vi "Teleop.vi"(10 "Match Info":T1={"Autonomous Elapsed Seconds"=0.0, "TeleOp Elapsed Seconds"=0.0, "Disabled Elapsed Seconds"=0.0, "Visited Autonomous"=FALSE, "Visited TeleOp"=FALSE, "Visited Disabled"=FALSE, "Autonomous Settings"={"Autonomous Style"=enum."Independent", "VI Refnum"=refnum}}, 11 "Call Context":T2) -> ()   [LabVIEW 2018]
doc: "This VI is called for each TeleOp packet received from the DS where the robot is not disabled. It is often used to read from the joysticks and update I/O or to update setpoints for timed control loops. It should complete and return within 20 milliseconds or it may miss DS packets."
uses:
  <vilib>/Rock Robotics/WPI/DriverStation/WPI_DriverStationDerivedRobotMode.ctl
  <vilib>/Rock Robotics/WPI/DriverStation/WPI_DriverStationMatch Info.ctl
  <vilib>/Rock Robotics/WPI/ThirdParty/Phoenix-LabVIEW/Motor Controller/Controls/CTRE_Phoenix_MotorControl_ControlMode.ctl
  <vilib>/Rock Robotics/WPI/Solenoid/WPI_SolenoidValue.ctl
  <vilib>/Rock Robotics/WPI/Utilities/WPI_GetSetVariantRefNum.vi
  <vilib>/Rock Robotics/Network Tables/NT Write Numeric Array.vi
  <vilib>/Rock Robotics/Network Tables/NT Read Boolean.vi
  <vilib>/Rock Robotics/Network Tables/NT Read Number.vi
  <vilib>/Rock Robotics/WPI/Solenoid/WPI_SolenoidSetEnum.vi
panel:
  out "Sample Slider 0":dbl(slide) scale=0.0..5.0
  out "Sample Boolean 1":bool
  out "Sample Boolean 0":bool
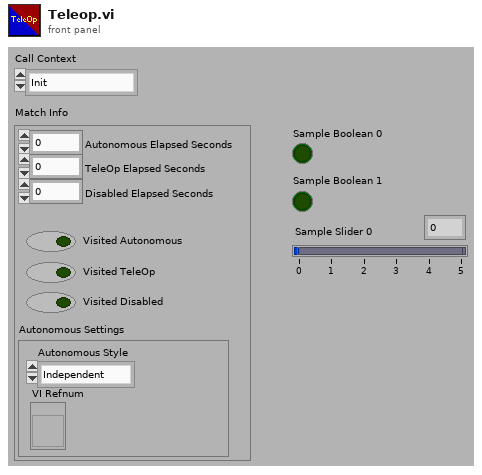
[diagram p1: front panel]
types:
  T1 = typedef "WPI_DriverStationMatch Info.ctl" = cluster{"Autonomous Elapsed Seconds":dbl, "TeleOp Elapsed Seconds":dbl, "Disabled Elapsed Seconds":dbl, "Visited Autonomous":bool, "Visited TeleOp":bool, "Visited Disabled":bool, "Autonomous Settings":cluster{"Autonomous Style":enum16{"Iterative", "Independent"}, "VI Refnum":refnum<vi>}}
  T2 = typedef "WPI_DriverStationDerivedRobotMode.ctl" = enum16{"Init", "Execute", "Stop"}
  T3 = typedef "CTRE_Phoenix_MotorControl_ControlMode.ctl" = u16
  T4 = typedef "WPI_JoystickDevRef.ctl" = cluster{"Device":T5}
  T5 = typedef "WPI_JoystickDeviceEnum.ctl" = enum16{"USB 0", "USB 1", "USB 2", "USB 3", "USB 4", "USB 5"}
  T6 = typedef "WPI_ServoDeviceRef.ctl" = cluster{"DeviceStatus":errorcluster, "PWM Channel":T7, "DeadBand":T8}
  T7 = typedef "FPGA_DIOPWMChannel.ctl" = enum8{"PWM 0", "PWM 1", "PWM 2", "PWM 3", "PWM 4", "PWM 5", "PWM 6", "PWM 7", "PWM 8", "PWM 9", "PWM MXP 0", "PWM MXP 1", "PWM MXP 2", "PWM MXP 3", "PWM MXP 4", "PWM MXP 5", "PWM MXP 6", "PWM MXP 7", "PWM MXP 8", "PWM MXP 9", "Invalid"}
  T8 = typedef "WPI_PWMDeadband.ctl" = cluster{"Name":string, "maxPositivePwm":i32, "minPositivePwm":i32, "centerPwm":i32, "maxNegativePwm":i32, "minNegativePwm":i32, "angularRange":u16}
  T9 = typedef "WPI_SolenoidDevRef.ctl" = cluster{"DevStatus":errorcluster, "Pneumatics Control Module":u8, "Forward Solenoid Channel":T10, "Reverse Solenoid Channel":T10}
  T10 = typedef "WPI_SolenoidChannel.ctl" = enum8{"Solenoid 0", "Solenoid 1", "Solenoid 2", "Solenoid 3", "Solenoid 4", "Solenoid 5", "Solenoid 6", "Solenoid 7", "Invalid"}
  T11 = typedef "WPI_RobotDriveDevRef.ctl" = cluster{"DevStatus":errorcluster, "Motors[]":T12[], "Square Inputs":bool, "Max Output":dbl}
  T12 = typedef "WPI_MotorControlDeviceRef.ctl" = cluster{"DeviceStatus":errorcluster, "Type":T13, "PWM":cluster{"PWM Channel":T7, "DeadBand":T8}, "CAN":cluster{"Device Number":u8, "SetOutput VI Ref":variant, "GetOutput VI Ref":variant, "Enable VI Ref":variant, "Disable VI Ref":variant, "Data":variant}, "Invert":bool, "DIO PWM":cluster{"PWM \"Enable\" Channel":T7, "DIOChannel":T14, "PWM Rate":dbl}}
  T13 = typedef "WPI_MotorControlType.ctl" = enum16{"PWM", "CAN", "DIO PWM"}
  T14 = typedef "FPGA_DIOChannel.ctl" = enum8{"DIO 0", "DIO 1", "DIO 2", "DIO 3", "DIO 4", "DIO 5", "DIO 6", "DIO 7", "DIO 8", "DIO 9", "DIO MXP 0", "DIO MXP 1", "DIO MXP 2", "DIO MXP 3", "DIO MXP 4", "DIO MXP 5", "DIO MXP 6", "DIO MXP 7", "DIO MXP 8", "DIO MXP 9", "DIO MXP 10", "DIO MXP 11", "DIO MXP 12", "DIO MXP 13", "DIO MXP 14", "DIO MXP 15", "SPI Port CS1", "SPI Port CS2", "SPI Port CS3", "SPI Port MISO", "SPI Port MOSI", "Invalid"}
  T15 = typedef "WPI_DigitalInputDevRef.ctl" = cluster{"DevStatus":errorcluster, "DIO Channel":T14}
  T16 = typedef "WPI_SolenoidValue.ctl" = enum16{"Off", "On", "Forward", "Reverse"}
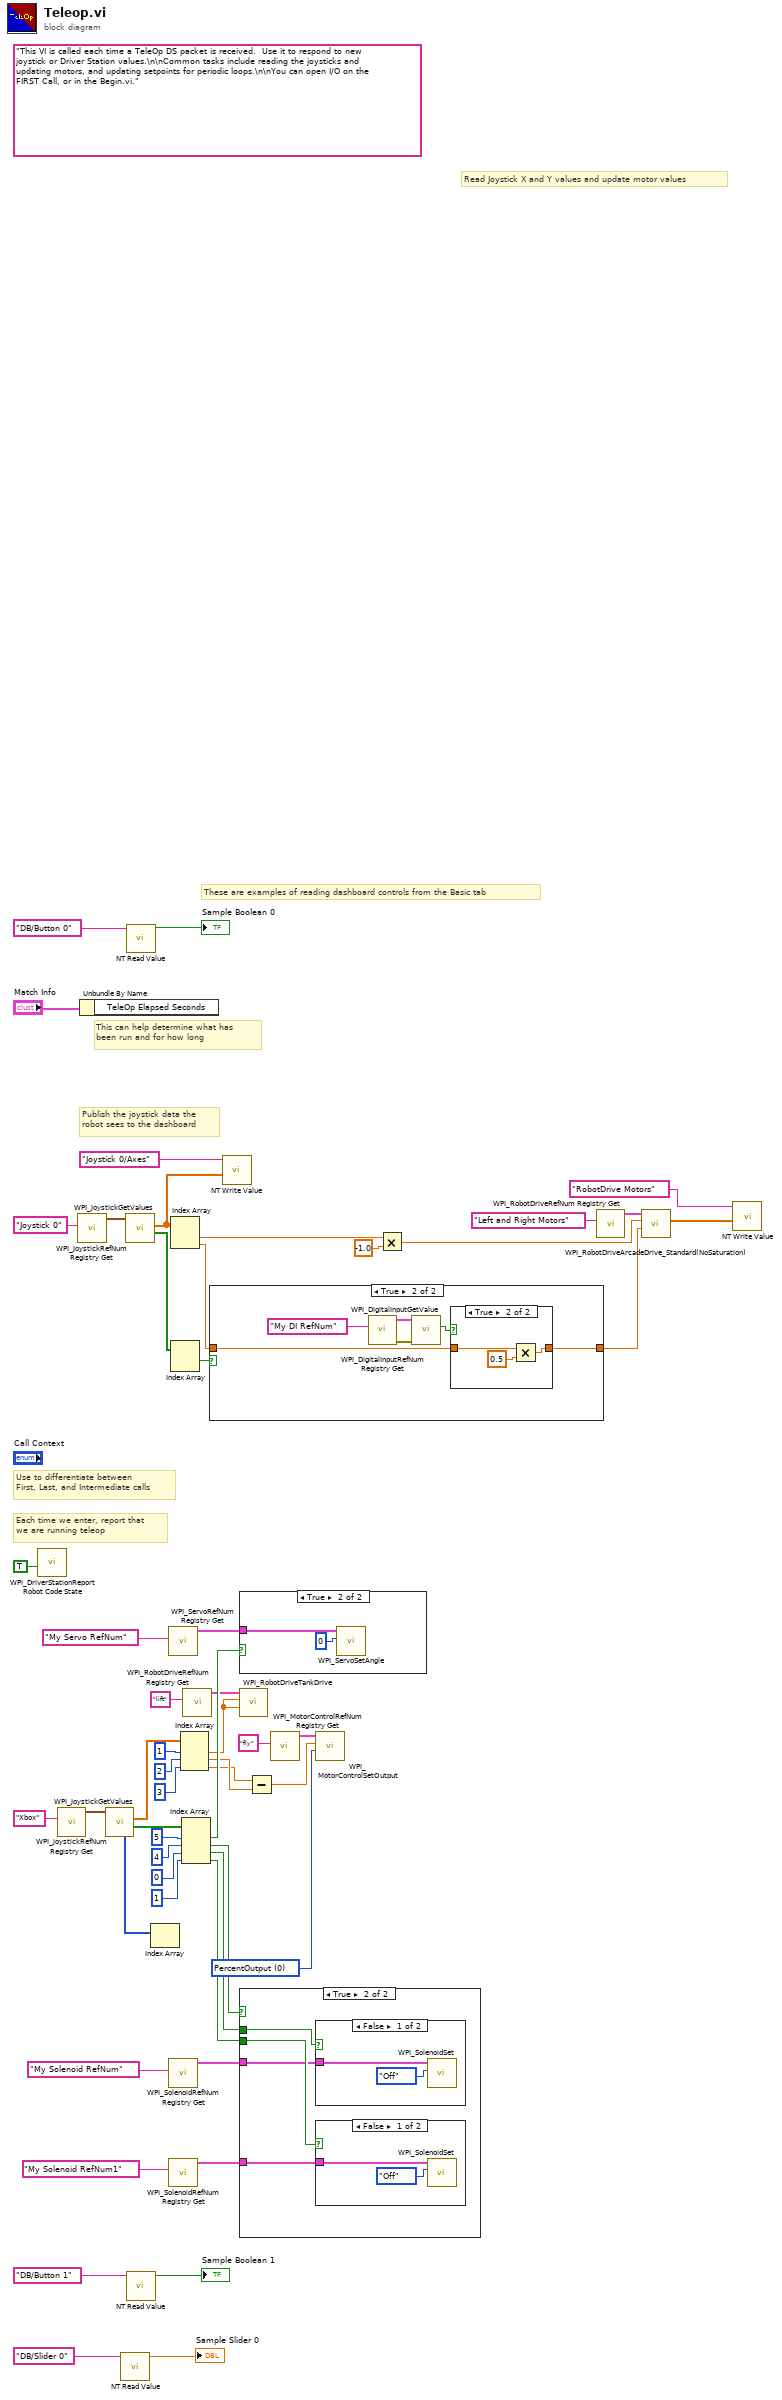
[diagram p0: block diagram]
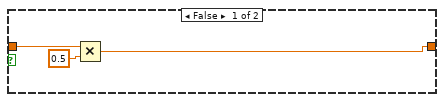
[diagram p2: hidden frame]
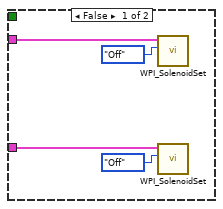
[diagram p4: hidden frame]
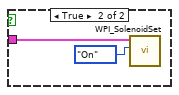
[diagram p5: hidden frame]
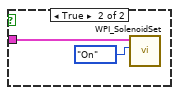
[diagram p6: hidden frame]
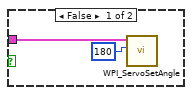
[diagram p7: hidden frame]
diagram:
  w11 = T3 0 items=["PercentOutput"=0, "Position"=1, "Velocity"=2, "Current"=3, "Follower"=5, "MotionProfile"=6, "MotionMagic"=7, "MotionProfileArc"=10, "Disabled"=15] ("Control Mode")
  (unwired) "This VI is called each time a TeleOp DS packet is received.  Use it to respond to new joystick or Driver Station values.\n\nCommon tasks include reading the joysticks and updating motors, and updating setpoints for periodic loops.\n\nYou can open I/O on the FIRST Call, or in the Begin.vi."
  # "These are examples of reading dashboard controls from the Basic tab"
  # "Publish the joystick data the\nrobot sees to the dashboard"
  # "Each time we enter, report that\nwe are running teleop"
  # "Use to differentiate between\nFirst, Last, and Intermediate calls"
  # "This can help determine what has\nbeen run and for how long"
  # "Read Joystick X and Y values and update motor values"
  n1 = call <vilib>:"WPI_DriverStationReport Robot Code State.vi"("TeleOp"=TRUE ("Autonomous")) -> ()  [unwired: 10 in, 1 out]
  n2 = call <vilib>:"WPI_JoystickRefNum Registry Get.vi"("refnum name"="Xbox") -> ("JoystickDevRef"=w37:T4)  [unwired: 1 in, 9 out]
  n3 = call <vilib>:"WPI_JoystickRefNum Registry Get.vi"("refnum name"="Joystick 0") -> ("JoystickDevRef"=w50:T4)  [unwired: 1 in, 9 out]
  n4 = Unbundle By Name("Match Info") -> ()  [unwired: 1 out]
  n5 = call <vilib>:"WPI_JoystickGetValues.vi"("JoystickDevRef"=w37) -> ("Buttons"=w36:bool[], "Axes"=w22:dbl[], "POVs"=w8:i16[])  [unwired: 6 in, 2 out]
  n6 = call-poly <vilib>:"NT Read Value.vi"("Name"="DB/Slider 0" ("refnum name")) -> ("Numeric"=→"Sample Slider 0":dbl)  [unwired: 9 in, 1 out]
  n7 = call <vilib>:"WPI_JoystickGetValues.vi"("JoystickDevRef"=w50) -> ("Buttons"=w7:bool[], "Axes"=w47:dbl[])  [unwired: 6 in, 3 out]
  n8 = call-poly <vilib>:"NT Read Value.vi"("Name"="DB/Button 0" ("refnum name")) -> ("Boolean"=→"Sample Boolean 0":bool)  [unwired: 9 in, 1 out]
  n9 = call-poly <vilib>:"NT Read Value.vi"("Name"="DB/Button 1" ("refnum name")) -> ("Boolean"=→"Sample Boolean 1":bool)  [unwired: 9 in, 1 out]
  n10 = Index Array(array=w8) -> ()  [unwired: 1 in, 1 out]
  n11 = call <vilib>:"WPI_ServoRefNum Registry Get.vi"("refnum name"="My Servo RefNum") -> ("ServoDeviceRef"=w33:T6)  [unwired: 9 in, 1 out]
  n12 = call <vilib>:"WPI_SolenoidRefNum Registry Get.vi"("refnum name"="My Solenoid RefNum") -> ("SolenoidDevRef"=w30:T9)  [unwired: 9 in, 1 out]
  n13 = call <vilib>:"WPI_SolenoidRefNum Registry Get.vi"("refnum name"="My Solenoid RefNum1") -> ("SolenoidDevRef"=w24:T9)  [unwired: 9 in, 1 out]
  n14 = Index Array(array=w47) -> (element #1=w3:dbl, element #2=w4:dbl)  [unwired: 2 in]
  n15 = Index Array(array=w7) -> (element #1=w6:bool)  [unwired: 2 in, 1 out]
  n16 = Index Array(array=w22, index #1=1 ("index"), index #2=2 ("index"), index #3=3 ("index")) -> (element #1=w19:dbl, element #2=w16:dbl, element #3=w15:dbl)
  n17 = Index Array(array=w36, index #1=5 ("index"), index #2=4 ("index"), index #3=0 ("index"), index #4=1 ("index")) -> (element #1=w34:bool, element #2=w28:bool, element #3=w10:bool, element #4=w9:bool)
  n18 = call <vilib>:"WPI_RobotDriveRefNum Registry Get.vi"("refnum name"="lift") -> ("RobotDriveDevRef"=w18:T11)  [unwired: 9 in, 1 out]
  n19 = case shown="True" w6 {
    tunnel: w4 -> [w56 w63]
    tunnel: [w55 w62] -> w5
    frame False {
      n20 = Multiply(x=w56, y=0.5) -> (x*y=w55:dbl)
    }
    frame True {
      n21 = call <vilib>:"WPI_DigitalInputRefNum Registry Get.vi"("refnum name"="My DI RefNum") -> ("error out"=w60:errorcluster, "DigitalInputDevRef"=w61:T15)  [unwired: 9 in]
      n22 = call <vilib>:"WPI_DigitalInputGetValue.vi"("error in (no error)"=w60, "DigitalInputDevRef"=w61) -> ("Value"=w58:bool)  [unwired: 7 in, 2 out]
      n23 = case shown="True" w58 {
        tunnel: w63 -> [w64 w66]
        tunnel: [w64 w65] -> w62
        frame False {
        }
        frame True {
          n24 = Multiply(x=w66, y=0.5) -> (x*y=w65:dbl)
        }
      }
    }
  }
  n25 = call-poly <vilib>:"NT Write Value.vi"("Numeric Array"=w47, "Name"="Joystick 0/Axes") -> ()  [unwired: 9 in, 1 out]
  n26 = case shown="True" w34 {
    tunnel: w33 -> [w68 w71]
    frame False {
      n27 = call <vilib>:"WPI_ServoSetAngle.vi"("Angle"=180, "ServoDeviceRef"=w68) -> ()  [unwired: 8 in, 2 out]
    }
    frame True {
      n28 = call <vilib>:"WPI_ServoSetAngle.vi"("Angle"=0, "ServoDeviceRef"=w71) -> ()  [unwired: 8 in, 2 out]
    }
  }
  n29 = call <vilib>:"WPI_RobotDriveTankDrive.vi"("Right axis value"=w19, "Left axis value"=w19, "RobotDriveDevRef"=w18) -> ()  [unwired: 6 in, 3 out]
  n30 = case shown="True" w28 {
    tunnel: w30 -> [w74 w76]
    tunnel: w24 -> [w72 w77]
    tunnel: w10 -> [_ w79]
    tunnel: w9 -> [_ w78]
    frame False {
      n31 = call-poly <vilib>:"WPI_SolenoidSet.vi"("Value"=WPI_SolenoidValue."Off", "SolenoidDevRef"=w74) -> ()  [unwired: 8 in, 2 out]
      n32 = call-poly <vilib>:"WPI_SolenoidSet.vi"("Value"=WPI_SolenoidValue."Off", "SolenoidDevRef"=w72) -> ()  [unwired: 8 in, 2 out]
    }
    frame True {
      n33 = case shown="False" w79 {
        tunnel: w76 -> [w84 w87]
        frame False {
          n34 = call-poly <vilib>:"WPI_SolenoidSet.vi"("Value"=WPI_SolenoidValue."Off", "SolenoidDevRef"=w84) -> ()  [unwired: 8 in, 2 out]
        }
        frame True {
          n35 = call-poly <vilib>:"WPI_SolenoidSet.vi"("Value"=WPI_SolenoidValue."On", "SolenoidDevRef"=w87) -> ()  [unwired: 8 in, 2 out]
        }
      }
      n36 = case shown="False" w78 {
        tunnel: w77 -> [w80 w83]
        frame False {
          n37 = call-poly <vilib>:"WPI_SolenoidSet.vi"("Value"=WPI_SolenoidValue."Off", "SolenoidDevRef"=w80) -> ()  [unwired: 8 in, 2 out]
        }
        frame True {
          n38 = call-poly <vilib>:"WPI_SolenoidSet.vi"("Value"=WPI_SolenoidValue."On", "SolenoidDevRef"=w83) -> ()  [unwired: 8 in, 2 out]
        }
      }
    }
  }
  n39 = Subtract(x=w15, y=w16) -> (x-y=w12:dbl)
  n40 = call <vilib>:"WPI_MotorControlRefNum Registry Get.vi"("refnum name"="fly") -> ("MotorControlDevRef"=w14:T12)  [unwired: 9 in, 1 out]
  n41 = call <vilib>:"WPI_MotorControlSetOutput.vi"("options"=w11, "Output"=w12, "MotorControlDevRef"=w14) -> ()  [unwired: 6 in, 3 out]
  n42 = Multiply(x=w3, y=-1.0) -> (x*y=w2:dbl)
  n43 = call <vilib>:"WPI_RobotDriveRefNum Registry Get.vi"("refnum name"="Left and Right Motors") -> ("RobotDriveDevRef"=w52:T11)  [unwired: 1 in, 9 out]
  n44 = call <vilib>:"WPI_RobotDriveArcadeDrive_Standard(NoSaturation).vi"("Y axis value"=w5, "X axis value"=w2, "RobotDriveDevRef"=w52) -> ("Motor Values"=w40:dbl[])  [unwired: 1 in, 7 out]
  n45 = call-poly <vilib>:"NT Write Value.vi"("Numeric Array"=w40, "Name"="RobotDrive Motors") -> ()  [unwired: 9 in, 1 out]
